vi "Vision Server Clear Vision Updates.vi"(1 "Vision Server":T1) -> (0 "Vision Server":T1)   [LabVIEW 2016]
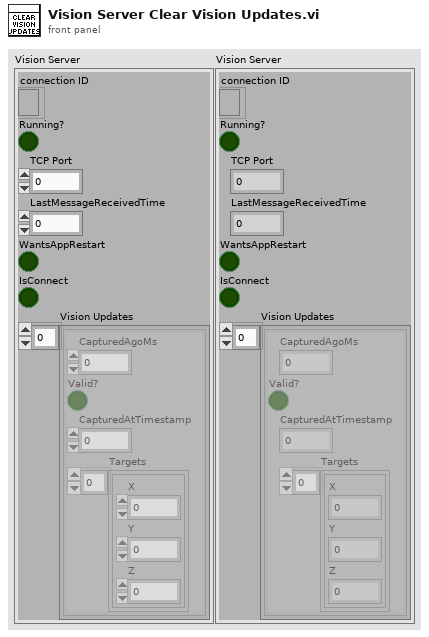
[diagram p1: front panel]
types:
  T1 = cluster{"connection ID":refnum<k5>, "Running?":bool, "TCP Port":u16, "LastMessageReceivedTime":dbl, "WantsAppRestart":bool, "IsConnect":bool, "Vision Updates":cluster{"CapturedAgoMs":i32, "Valid?":bool, "CapturedAtTimestamp":dbl, "Targets":cluster{"X":dbl, "Y":dbl, "Z":dbl}[]}[]}
  T2 = cluster{"CapturedAgoMs":i32, "Valid?":bool, "CapturedAtTimestamp":dbl, "Targets":cluster{"X":dbl, "Y":dbl, "Z":dbl}[]}[]
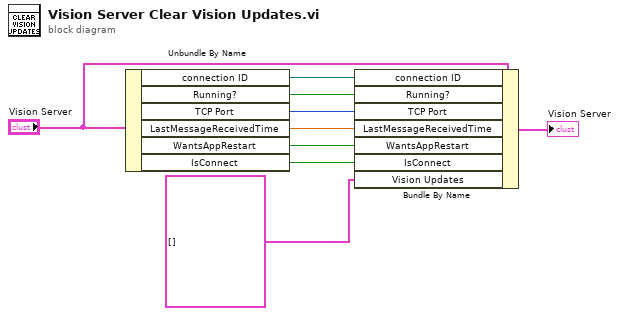
[diagram p0: block diagram]
diagram:
  n1 = Unbundle By Name("Vision Server") -> ("connection ID"=w9:refnum<k5>, "Running?"=w8:bool, "TCP Port"=w7:u16, "LastMessageReceivedTime"=w6:dbl, "WantsAppRestart"=w5:bool, "IsConnect"=w4:bool)
  n2 = Bundle By Name(cluster="Vision Server", "connection ID"=w9, "Running?"=w8, "TCP Port"=w7, "LastMessageReceivedTime"=w6, "WantsAppRestart"=w5, "IsConnect"=w4, "Vision Updates"=T2 []) -> (→"Vision Server":T1)
